vi "RANGE ANSI Message.vi"(10 "Bank Counter":i32, 11 "Count Down Timer":i32) -> (3 "ANSI Display 3":string)   [LabVIEW 2016]
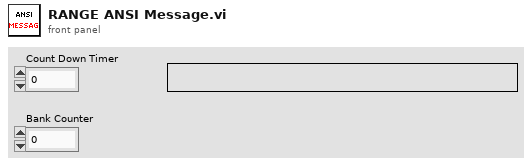
[diagram p1: front panel]
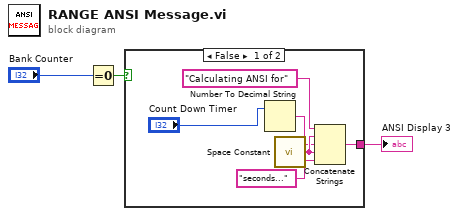
[diagram p0: block diagram]
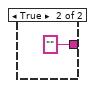
[diagram p2: hidden frame]
diagram:
  n1 = Equal To 0?(x="Bank Counter") -> (x = 0?=w1:bool)
  n2 = case shown="False" w1 {
    tunnel: [w9 ""] -> w3
    frame False {
      n3 = Number To Decimal String(number="Count Down Timer") -> (decimal integer string=w6:string)  [unwired: 1 in]
      n4 = call <vilib>:"Space Constant.vi"() -> ("String"=w7:string)
      n5 = Concatenate Strings("Calculating ANSI for", w7, w6, w7, "seconds..." ("string")) -> (w9:string)
    }
    frame True {
    }
  }
  "ANSI Display 3" <- w3
